vi "S3859061_Task1.vi"() -> ()   [LabVIEW 2020]
panel:
  out "distance":dbl
  in  "y2":dbl
  in  "x2":dbl
  in  "y1":dbl
  in  "x1":dbl
  in  "stop":bool
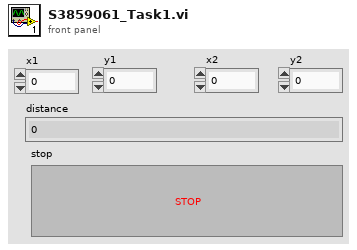
[diagram p1: front panel]
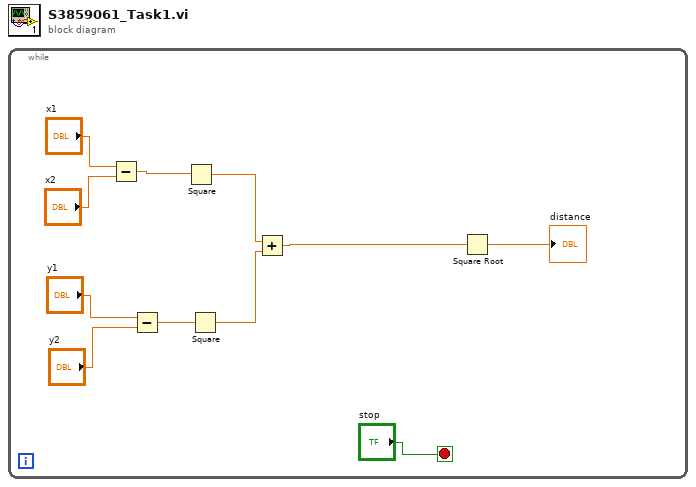
[diagram p0: block diagram]
diagram:
  n1 = while {
    stop <- "stop" stop-if-true
    n2 = Subtract(x="x1", y="x2") -> (x-y=w6:dbl)
    n3 = Subtract(x="y1", y="y2") -> (x-y=w5:dbl)
    n4 = Square(x=w6) -> (x^2=w4:dbl)
    n5 = Square(x=w5) -> (x^2=w3:dbl)
    n6 = Add(x=w4, y=w3) -> (x+y=w2:dbl)
    n7 = Square Root(x=w2) -> (sqrt(x)=→"distance":dbl)
  }
